vi "Combine Into Array Into One Sequence.vi"(1 "Array of Seqs in":refnum<class "Sequence of SBlocks.lvclass">[](array[class])) -> (0 "Array of Seqs out":refnum<class "Sequence of SBlocks.lvclass">[](array[class]))   [LabVIEW 2020, in "TALOS.lvlib" / "Scheduler.lvlib" / "Scheduler.lvclass"]
uses:
  Scheduler.lvclass
  Run Utilities/Sequence of SBlocks/Sequence of SBlocks.lvclass
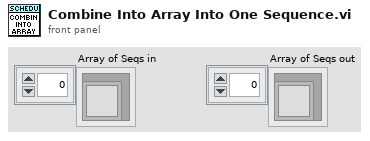
[diagram p1: front panel]
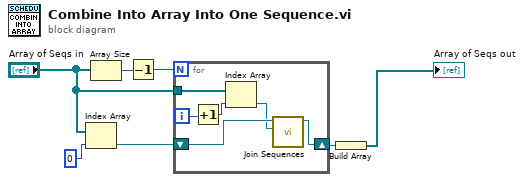
[diagram p0: block diagram]
diagram:
  n1 = Index Array(array="Array of Seqs in", index=0) -> (element=w2:refnum<class "Sequence of SBlocks.lvclass">)
  n2 = Array Size(array="Array of Seqs in") -> (size(s)=w6:i32)
  n3 = Decrement(x=w6) -> (x-1=w7:i32)
  n4 = for {
    N: w7 -> [_]
    shift-right: [w10] -> w4
    shift-left: w2 -> [w9]
    tunnel: "Array of Seqs in" -> [w13]
    i -> [w12]
    n5 = Increment(x=w12) -> (x+1=w11:i32)
    n6 = Index Array(array=w13, index=w11) -> (element=w8:refnum<class "Sequence of SBlocks.lvclass">)
    n7 = call-dynamic "Join Sequences.vi"("Sequence of SBlocks"=w8, "Sequence of SBlocks in"=w9) -> ("Sequence of SBlocks out"=w10:refnum<class "Sequence of SBlocks.lvclass">)  [unwired: 8 in, 1 out]
  }
  n8 = Build Array(w4) -> (→"Array of Seqs out":refnum<class "Sequence of SBlocks.lvclass">[])
